vi "Default Implementation.vi"(10 "Implementation":refnum<class>) -> (2 "Default Implementation":refnum<class>)   [LabVIEW 2020, in "jettl.lvlib"]
uses:
  jettl.lvlib
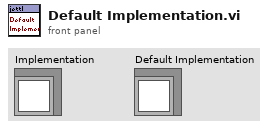
[diagram p1: front panel]
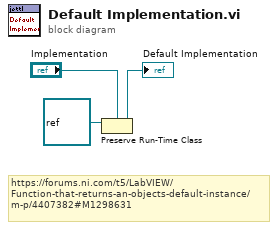
[diagram p0: block diagram]
diagram:
  # "https://forums.ni.com/t5/LabVIEW/Function-that-returns-an-objects-default-instance/m-p/4407382#M1298631"
  n1 = Preserve Run-Time Class(object in=refnum<class> refnum ("LabVIEW Object"), 2:"Implementation") -> (object out=→"Default Implementation":refnum<class>)  [unwired: 1 in, 1 out]
